vi "Set IVirtual Instrument.vi"(10 "IVirtual Instrument":refnum<class "IVirtual Instrument.lvclass">, 11 "Action Point in":refnum<class "Action Point.lvclass">) -> (3 "Action Point out":refnum<class "Action Point.lvclass">)   [LabVIEW 2025]
uses:
  Action Point.lvclass/Action Point.ctl
  Action Point.lvclass
  D:/git/HAL/Source/Action Point/Action Point.lvclass
  D:/git/HAL/Source/Interfaces/IInitialize/IInitialize.lvclass
  Interfaces/IVirtual Instrument/IVirtual Instrument.lvclass
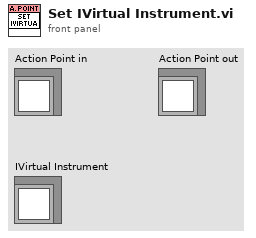
[diagram p1: front panel]
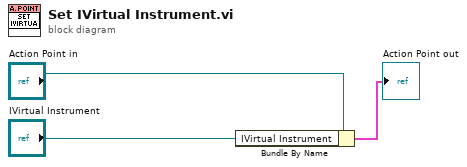
[diagram p0: block diagram]
diagram:
  n1 = Bundle By Name(cluster="Action Point in", "IVirtual Instrument"="IVirtual Instrument") -> (→"Action Point out":cluster{})
